vi "Show or Hide Normally Connected Endpoint Information.vi"(8 "error in (no error)":errorcluster, 10 "Main Page Controls":T2, 11 "ni-switch custom device in":T1 format="%.0x") -> (0 "error out":errorcluster, 3 "ni-switch custom device out":T1 format="%.0x")   [LabVIEW 2020, in "NI-SWITCH System Explorer.lvlib"]
uses:
  NI-SWITCH System Explorer.lvlib
  Main Page Controls.ctl
  <vilib>/NI VeriStand/Custom Device API/Custom Device Item Ref.ctl
  Shared/Routing and Faulting Hardware API/Routing and Faulting Hardware API.lvlib
  <vilib>/NI VeriStand/Custom Device API/Custom Device API.lvlib
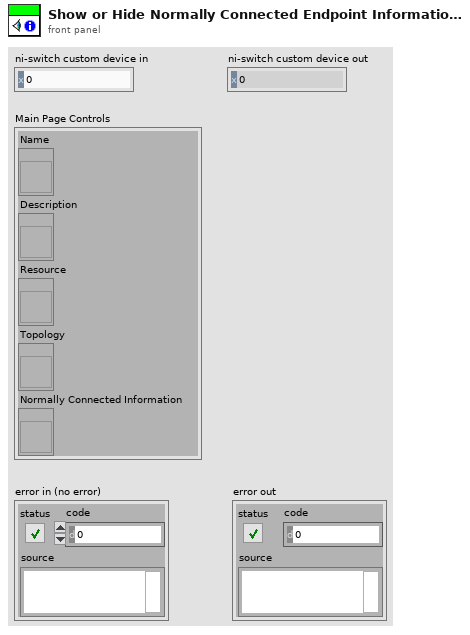
[diagram p1: front panel]
types:
  T1 = typedef "Custom Device API.lvlib/Custom Device Item Ref.ctl" = u64
  T2 = typedef "NI-SWITCH System Explorer.lvlib/Main Page Controls.ctl" = cluster{"Name":refnum<vi>, "Description":refnum<vi>, "Resource":refnum<vi>, "Topology":refnum<vi>, "Normally Connected Information":refnum<vi>}
  T3 = typedef "Routing and Faulting Hardware API.lvlib/Connection.ctl" = cluster{"Endpoint 1":string, "Endpoint 2":string}
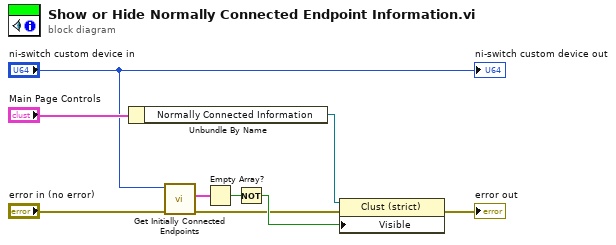
[diagram p0: block diagram]
diagram:
  n1 = Unbundle By Name("Main Page Controls") -> ("Normally Connected Information"=w7:refnum<vi>)
  n2 = call "Get Initially Connected Endpoints.vi"("error in (no error)"="error in (no error)", "Hardware Ref in"="ni-switch custom device in") -> ("error out"=w4:errorcluster, "Connections"=w3:T3[])  [unwired: 7 in, 1 out]
  n3 = Empty Array?(array=w3) -> (empty?=w8:bool)
  n4 = Not(x=w8) -> (.not. x?=w9:bool)
  n5 = property class="Clust (strict)"(reference=w7, error in=w4, "Visible"=w9) -> (error out=→"error out":errorcluster)  [unwired: 1 out]
  "ni-switch custom device out" <- "ni-switch custom device in"
